vi "Calculate Refactor Metrics for Project.vi"(5 "refactored labels":T1[](array[typedef]), 6 "refactored overrides":T5[](array[typedef]), 7 "refactored string constants":T1[](array[typedef]), 8 "error in":errorcluster, 9 "refactored classes":path[](array[path]), 10 "refactored dependencies":T6(array[cluster]), 11 "project path":path) -> (0 "error out":errorcluster, 3 "refactor result":T3)   [LabVIEW 2021, in "MeasurementService Editor.lvlib"]
uses:
  MeasurementService Editor.lvlib
  Refactor Object Result.ctl
  Refactor Dynamic Dispatch Member Result.ctl
  Refactor Project Result.ctl
  Rename String.ctl
  Rename String Result.ctl
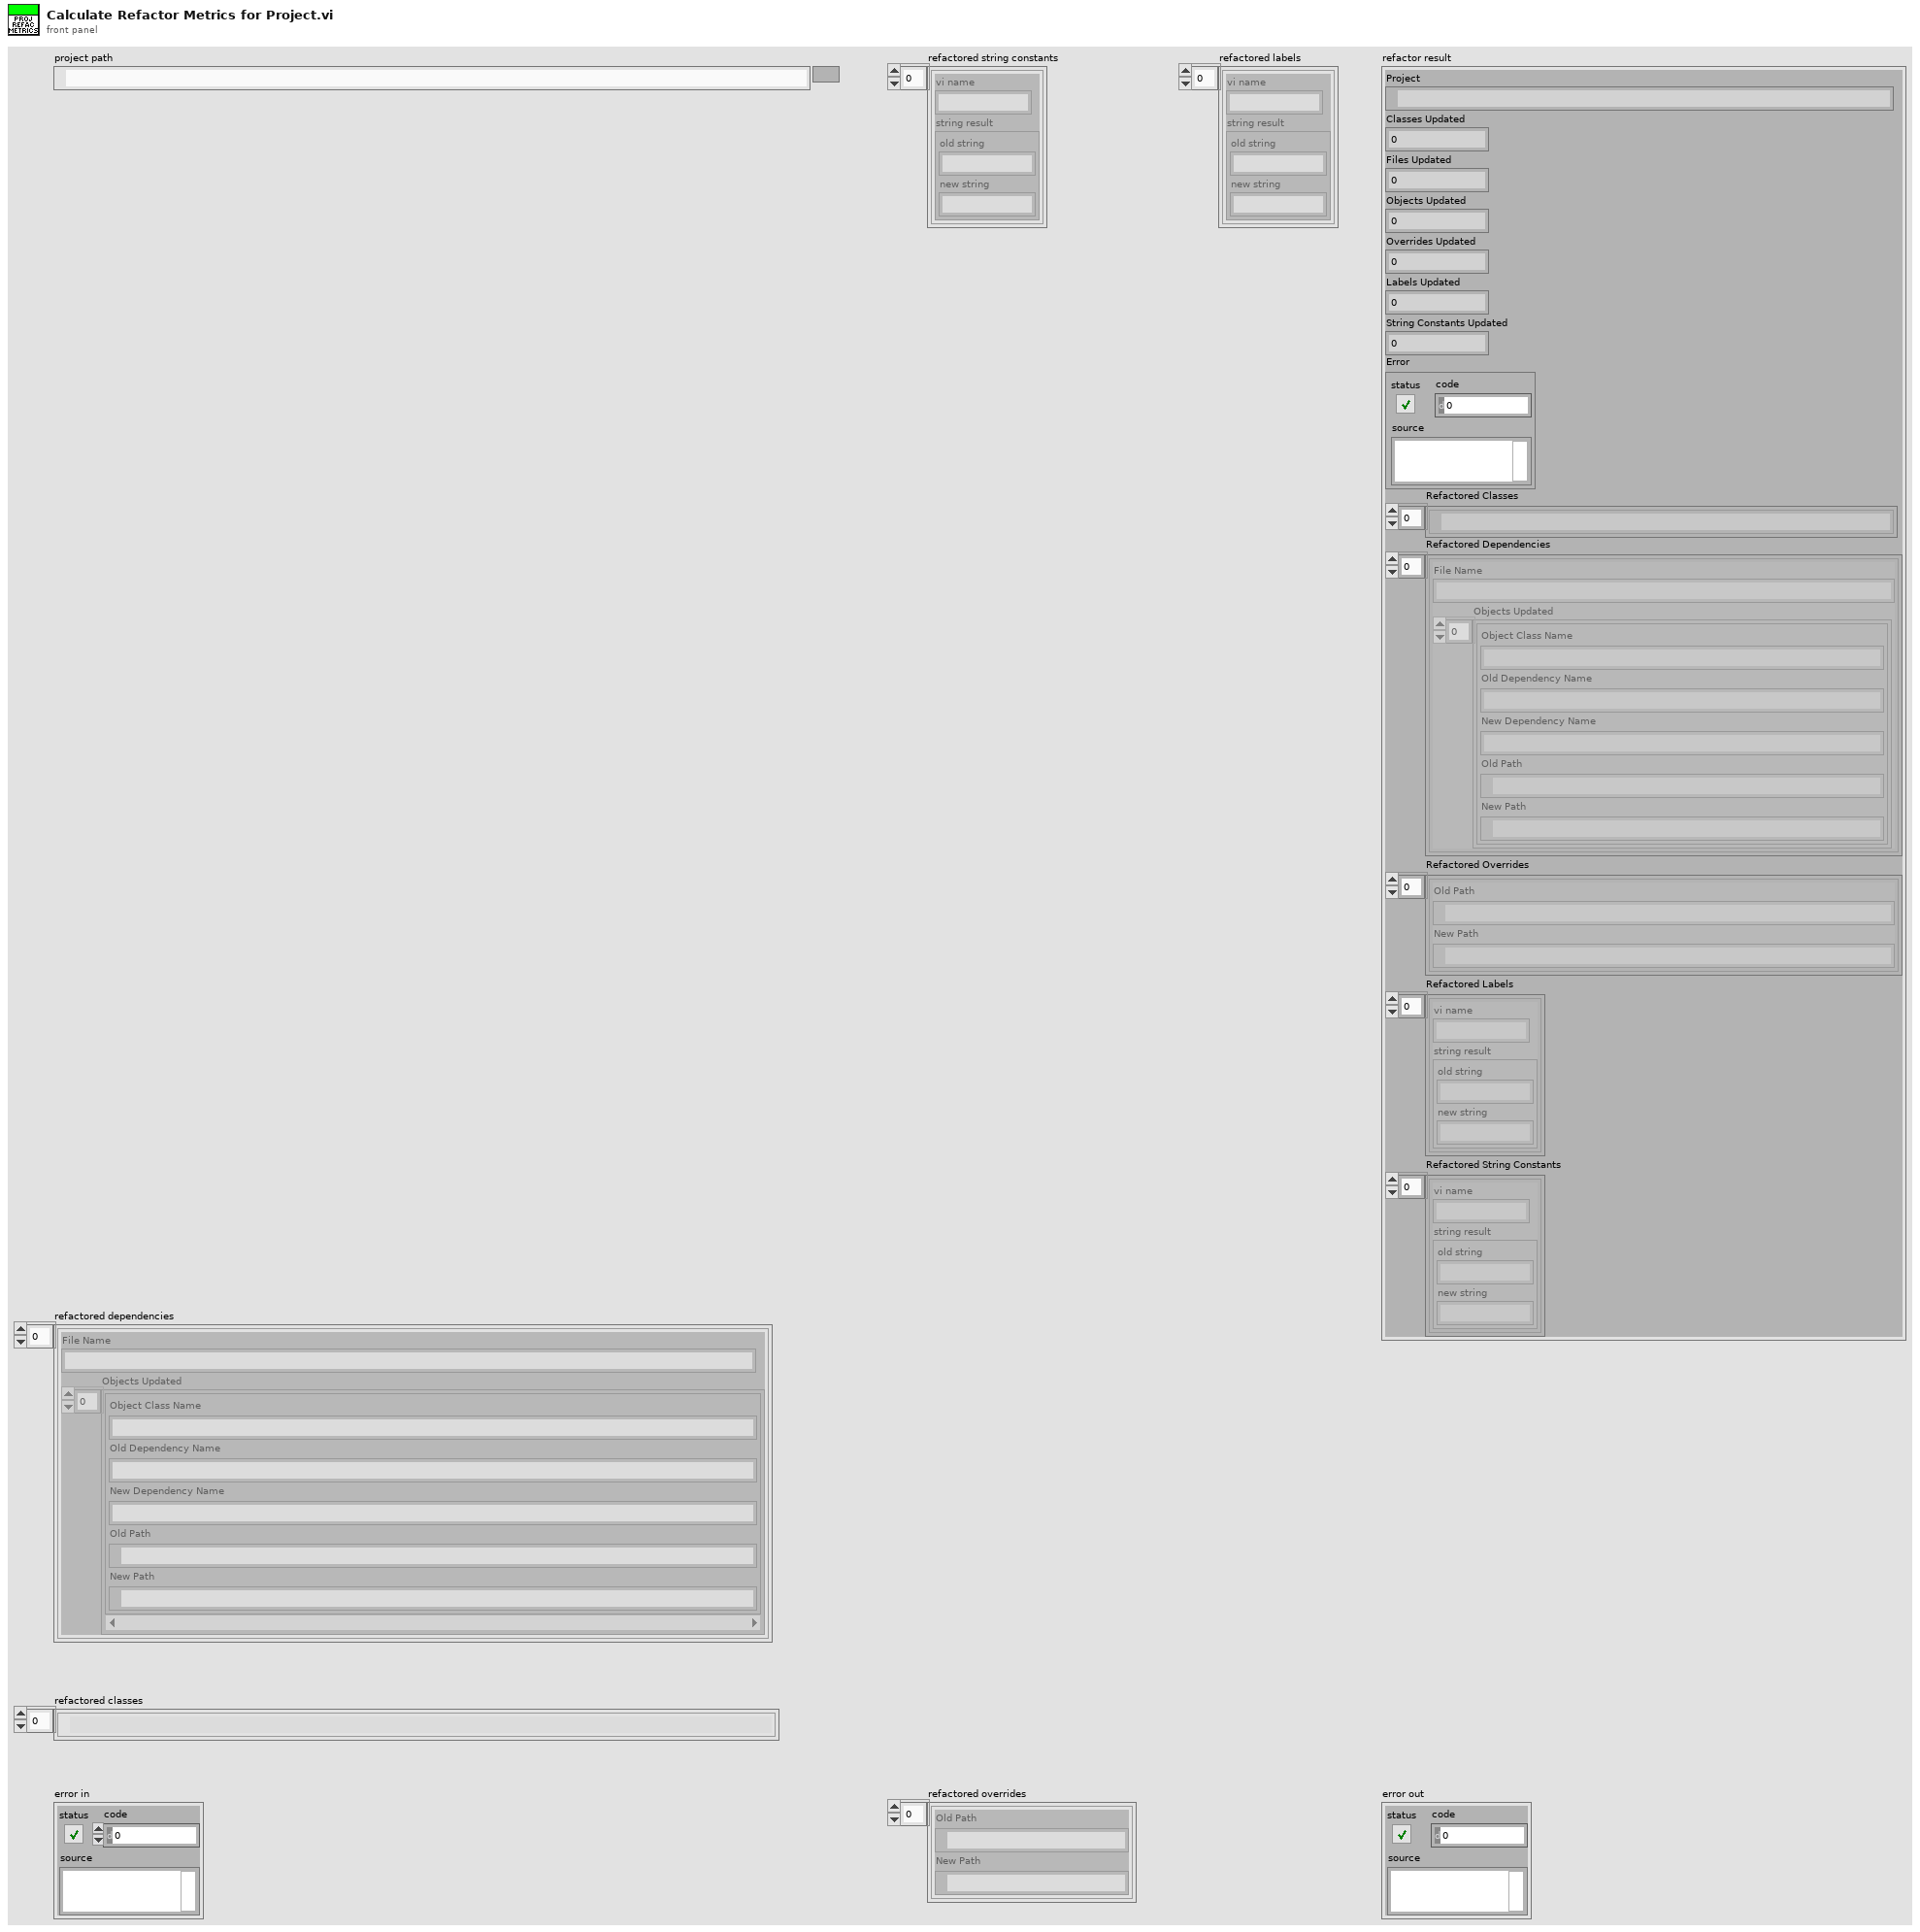
[diagram p1: front panel]
types:
  T1 = typedef "MeasurementService Editor.lvlib/Rename String Result.ctl" = cluster{"vi name":string, "string result":T2}
  T2 = typedef "MeasurementService Editor.lvlib/Rename String.ctl" = cluster{"old string":string, "new string":string}
  T3 = typedef "MeasurementService Editor.lvlib/Refactor Project Result.ctl" = cluster{"Project":path, "Classes Updated":u32, "Files Updated":u32, "Objects Updated":u32, "Overrides Updated":u32, "Labels Updated":u32, "String Constants Updated":u32, "Error":errorcluster, "Refactored Classes":path[], "Refactored Dependencies":cluster{"File Name":string, "Objects Updated":T4[]}[], "Refactored Overrides":T5[], "Refactored Labels":T1[], "Refactored String Constants":T1[]}
  T4 = typedef "MeasurementService Editor.lvlib/Refactor Object Result.ctl" = cluster{"Object Class Name":string, "Old Dependency Name":string, "New Dependency Name":string, "Old Path":path, "New Path":path}
  T5 = typedef "MeasurementService Editor.lvlib/Refactor Dynamic Dispatch Member Result.ctl" = cluster{"Old Path":path, "New Path":path}
  T6 = cluster{"File Name":string, "Objects Updated":T4[]}[]
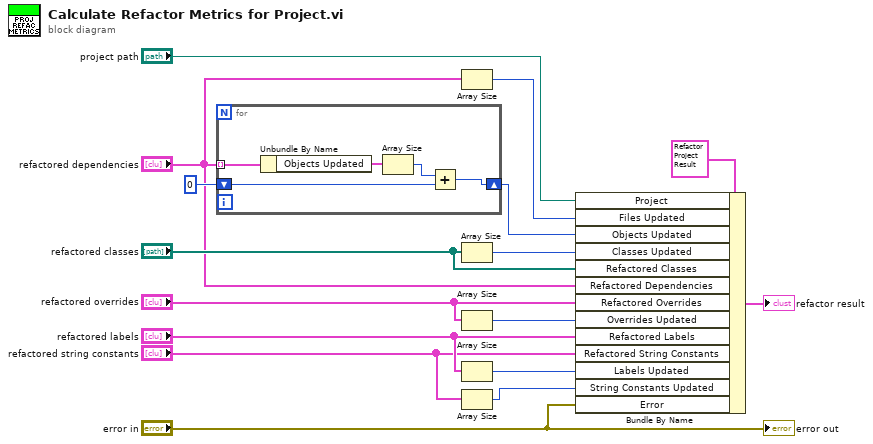
[diagram p0: block diagram]
diagram:
  n1 = for {
    tunnel: "refactored dependencies" -> [w21] mode=indexing
    shift-right: [w17] -> w11
    shift-left: 0 -> [w18]
    n2 = Unbundle By Name(w21) -> ("Objects Updated"=w20:T4[])
    n3 = Array Size(array=w20) -> (size(s)=w19:i32)
    n4 = Add(x=w19, y=w18) -> (x+y=w17:i32)
  }
  n5 = Array Size(array="refactored dependencies") -> (size(s)=w10:i32)
  n6 = Array Size(array="refactored classes") -> (size(s)=w12:i32)
  n7 = Array Size(array="refactored overrides") -> (size(s)=w7:i32)
  n8 = Array Size(array="refactored labels") -> (size(s)=w4:i32)
  n9 = Array Size(array="refactored string constants") -> (size(s)=w2:i32)
  n10 = Bundle By Name(cluster=T3 {"Project"=path "", "Classes Updated"=0, "Files Updated"=0, "Objects Updated"=0, "Overrides Updated"=0, "Labels Updated"=0, "String Constants Updated"=0, "Error"={"status"=FALSE, "code"=0, "source"=""}, "Refactored Classes"=[], "Refactored Dependencies"=[], "Refactored Overrides"=[], "Refactored Labels"=[], "Refactored String Constants"=[]} ("Refactor Project Result"), "Project"="project path", "Files Updated"=w10, "Objects Updated"=w11, "Classes Updated"=w12, "Refactored Classes"="refactored classes", "Refactored Dependencies"="refactored dependencies", "Refactored Overrides"="refactored overrides", "Overrides Updated"=w7, "Refactored Labels"="refactored labels", "Refactored String Constants"="refactored string constants", "Labels Updated"=w4, "String Constants Updated"=w2, "Error"="error in") -> (→"refactor result":T3)
  "error out" <- "error in"
